vi "Get SMO RC Type.vi"(8 "error in (no error)":errorcluster, 11 "Instrument in":refnum<class "Instrument.lvclass">) -> (0 "error out":errorcluster, 2 "Dependencies.RemoteControl":refnum<class "RemoteControl.lvclass">, 3 "Instrument out":refnum<class "Instrument.lvclass">)   [LabVIEW 2019, in "Instrument.lvclass"]
doc: "Override this VI to return the type of RemoteControl process used by your Instrument. The default is RemoteControl.ZMQ"
uses:
  Instrument.lvclass
  <userlib>/LevyLab/RemoteControl/RemoteControl/RemoteControl.lvclass
  <userlib>/LevyLab/RemoteControl/RemoteControl.ZMQ/RemoteControl.ZMQ.lvclass
  C:/Program Files (x86)/National Instruments/LabVIEW 2019/user.lib/LevyLab/RemoteControl/RemoteControl/RemoteControl.lvclass
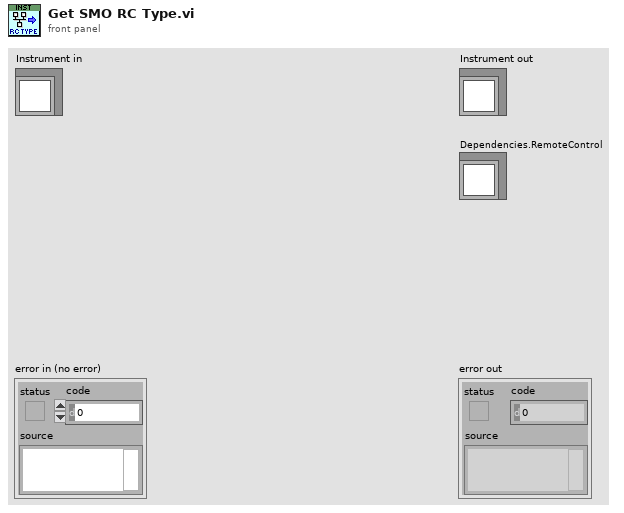
[diagram p1: front panel]
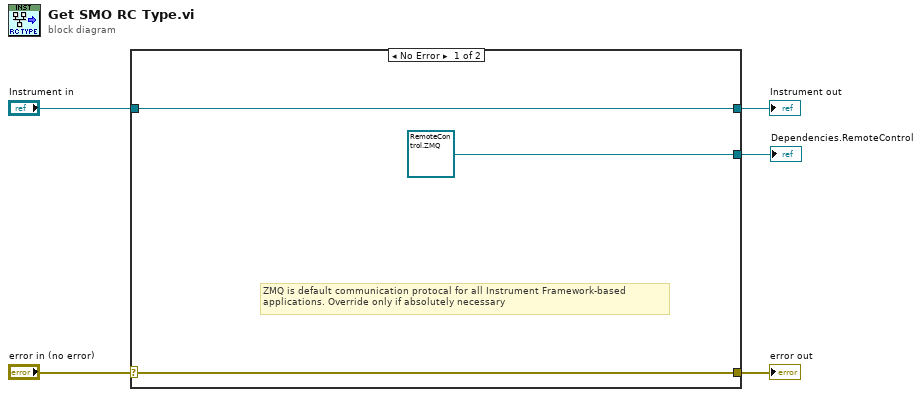
[diagram p0: block diagram]
diagram:
  n1 = case shown="No Error" "error in (no error)" {
    selector: "error in (no error)" -> [w8 w10]
    tunnel: [w8 w10] -> w4
    tunnel: [w7 w9] -> w2
    tunnel: "Instrument in" -> [w7 w9]
    tunnel: [refnum<class "RemoteControl.ZMQ.lvclass"> refnum ("RemoteControl.ZMQ.lvclass") _] -> w1
    frame No Error {
      # "ZMQ is default communication protocal for all Instrument Framework-based\napplications. Override only if absolutely necessary"
    }
    frame Error {
    }
  }
  "error out" <- w4
  "Instrument out" <- w2
  "Dependencies.RemoteControl" <- w1
